vi "New Log File Configuration.vi"(8 "error in (no error)":errorcluster, 9 "Default Log Directory":string[](array[string]), 10 "Default Name":string="Log File", 11 "Device Ref in":T1=18446744073709551615 format="%.0x") -> (0 "error out":errorcluster, 3 "Device Ref out":T1 format="%.0x")   [LabVIEW 2019, in "Telemetry System Explorer.lvlib"]
uses:
  Telemetry System Explorer.lvlib
  <vilib>/NI VeriStand/Custom Device API/Custom Device Item Ref.ctl
  Shared/Constants.vi
  <vilib>/NI VeriStand/Custom Device API/Set Item Property (String Array).vi
  <vilib>/NI VeriStand/Custom Device API/Set Item Property (Boolean).vi
  <vilib>/NI VeriStand/Custom Device API/Custom Device API.lvlib
  Shared/Telemetry Shared.lvlib
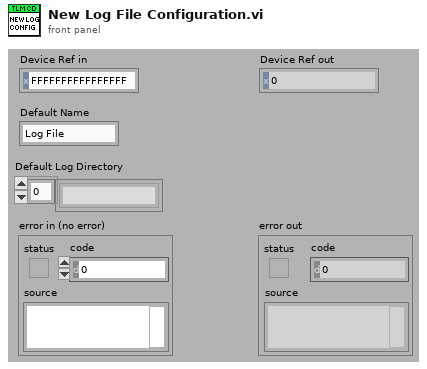
[diagram p1: front panel]
types:
  T1 = typedef "Custom Device API.lvlib/Custom Device Item Ref.ctl" = u64
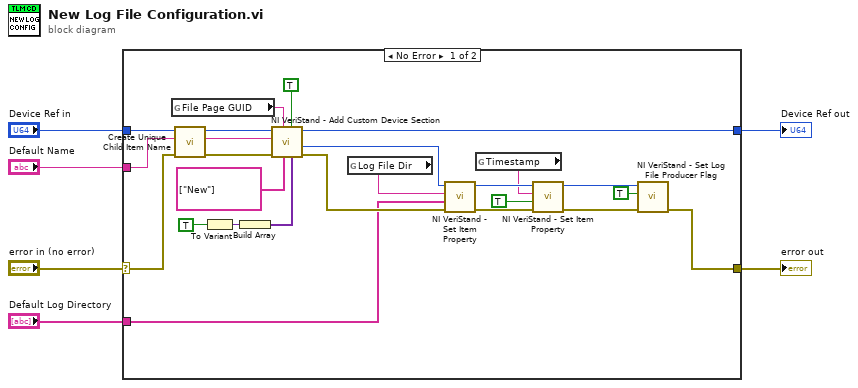
[diagram p0: block diagram]
diagram:
  n1 = case shown="No Error" "error in (no error)" {
    selector: "error in (no error)" -> [w19 w32]
    tunnel: "Default Name" -> [w30 _]
    tunnel: "Default Log Directory" -> [w10 _]
    tunnel: "Device Ref in" -> [w21 w33]
    tunnel: [w20 w33] -> w3
    tunnel: [w11 w32] -> w2
    frame No Error {
      n2 = global read "Constants.vi" "File Page GUID"() -> (w9:string)
      n3 = call "Create Unique Child Item Name.vi"("error in (no error)"=w19, "Name in"=w30, "Parent Item Ref in"=w21) -> ("error out"=w29:errorcluster, "Unique Name out"=w27:string, "Parent Item Ref out"=w28:T1)  [unwired: 6 in]
      n4 = To Variant(anything=TRUE) -> (Variant=w16:variant)
      n5 = Build Array(w16) -> (w15:variant[])
      n6 = call <vilib>:"NI VeriStand - Add Custom Device Section.vi"("Property Values"=w15, "Highlight? (F)"=TRUE, "Property names"=string[] ["New"], "GUID (Default Section)"=w9, "error in (no error)"=w29, "Section Name"=w27, "Parent Ref in"=w28) -> ("error out"=w31:errorcluster, "Section Ptr"=w22:T1, "Parent Ref out"=w20:T1)  [unwired: 2 out]
      n7 = global read "Constants.vi" "Log File Dir"() -> (w8:string)
      n8 = call-poly <vilib>:"NI VeriStand - Set Item Property.vi"("error in (no error)"=w31, "Value"=w10, "Property Name"=w8, "Item Ref in"=w22) -> ("error out"=w25:errorcluster, "Item Ref out"=w26:T1)  [unwired: 6 out]
      n9 = global read "Constants.vi" "Timestamp"() -> (w7:string)
      n10 = call-poly <vilib>:"NI VeriStand - Set Item Property.vi"("error in (no error)"=w25, "Value"=TRUE, "Property Name"=w7, "Item Ref in"=w26) -> ("error out"=w13:errorcluster, "Item Ref out"=w14:T1)  [unwired: 6 out]
      n11 = call <vilib>:"NI VeriStand - Set Log File Producer Flag.vi"("error in (no error)"=w13, "Log File Producer"=TRUE ("Log File Provider"), "Item Ref in"=w14) -> ("error out"=w11:errorcluster)  [unwired: 7 in, 1 out]
    }
    frame Error {
    }
  }
  "Device Ref out" <- w3
  "error out" <- w2
